vi "EllipseFitModule.vi"() -> ()   [LabVIEW 2011]
uses:
  Main/GlobalVariables.vi
panel:
  out "Valid Fit":bool
  in  "Reject Outliers":bool
  in  "bead":i32
  out "XY Graph bead 2":cluster{dbl[], dbl[]}[](graph)
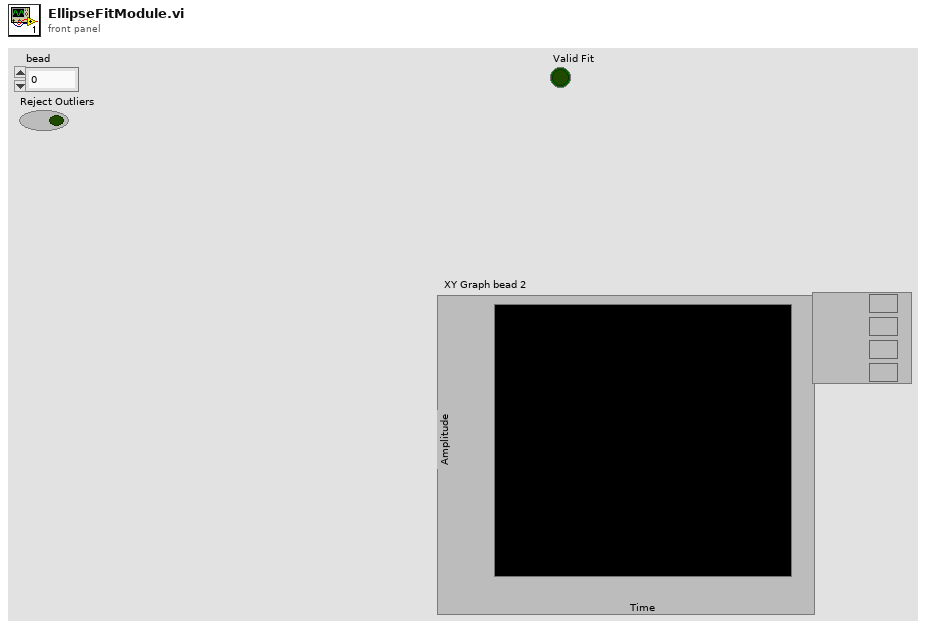
[diagram p1: front panel]
types:
  T1 = typedef "ResultManagerInstance.ctl" = cluster{"InstancePtr":u64}
  T2 = typedef "QTrkLocalizationResult.ctl" = cluster{"Queue Params":T3, "Position":T4, "Fast Estimate Position":cluster{"X":sgl, "Y":sgl}, "Error":i32, "Image mean":sgl}
  T3 = typedef "QTrkLocalizationJob.ctl" = cluster{"Frame#":u32, "Timestamp":u32, "ZLUT Index / bead#":i32, "Initial guess":T4}
  T4 = typedef "XYZf.ctl" = cluster{"X":sgl, "Y":sgl, "Z":sgl}
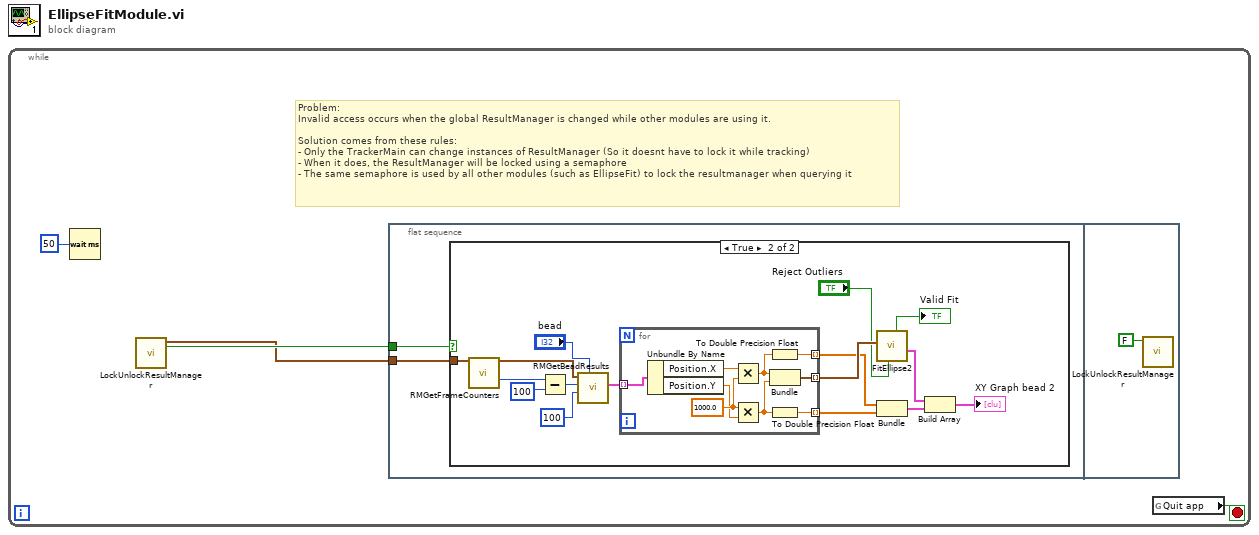
[diagram p0: block diagram]
diagram:
  n1 = while {
    stop <- w4 stop-if-true
    # "Problem: \nInvalid access occurs when the global ResultManager is changed while other modules are using it.\n\nSolution comes from these rules:\n- Only the TrackerMain can change instances of ResultManager (So it doesnt have to lock it while tracking)\n- When it does, the ResultManager will be locked using a semaphore\n- The same semaphore is used by all other modules (such as EllipseFit) to lock the resultmanager when querying it"
    n2 = Wait (ms)(milliseconds to wait=u32 50) -> ()  [unwired: 1 out]
    n3 = call "LockUnlockResultManager.vi"() -> ("Valid non-zero instance"=w2:bool, "ResultManager"=w1:T1)  [unwired: 9 in, 1 out]
    n4 = flat-sequence {
      tunnel: w2 -> [w6]
      tunnel: w1 -> [w5]
      frame #0 {
        n5 = case shown="True" w6 {
          tunnel: w5 -> [_ w22]
          frame False {
          }
          frame True {
            n6 = call "RMGetFrameCounters.vi"("ResultManager"=w22) -> ("ResultManager (out)"=w21:T1, "endFrame"=w20:i32)  [unwired: 7 in, 6 out]
            n7 = Subtract(x=w20, y=100) -> (x-y=w18:i32)
            n8 = call "RMGetBeadResults.vi"("bead"="bead", "numFrames"=100, "startFrame (0)"=w18, "ResultManager"=w21) -> ("results"=w15:T2[])  [unwired: 5 in, 2 out]
            n9 = for {
              tunnel: w15 -> [w31] mode=indexing
              tunnel: [w29] -> w14 mode=indexing
              tunnel: [w25] -> w7 mode=indexing
              tunnel: [w27] -> w8 mode=indexing
              w30 = sgl 1000.0 ("x")
              n10 = Unbundle By Name(w31) -> ("Position.X"=w26:sgl, "Position.Y"=w28:sgl)
              n11 = Multiply(x=w26, y=w30) -> (x*y=w24:sgl)
              n12 = Multiply(x=w30, y=w28) -> (x*y=w23:sgl)
              n13 = To Double Precision Float(number=w24) -> (double precision float=w25:dbl)
              n14 = Bundle(w24, w23) -> (w29:cluster{sgl, sgl})  [unwired: 1 in]
              n15 = To Double Precision Float(number=w23) -> (double precision float=w27:dbl)
            }
            n16 = call "FitEllipse2.vi"("Reject Outliers"="Reject Outliers", "Input data"=w14) -> ("XY Fit"=w11:cluster{dbl[], dbl[]}, "Valid Fit"=→"Valid Fit":bool)  [unwired: 7 in, 1 out]
            n17 = Bundle(w7, w8) -> (w10:cluster{dbl[], dbl[]})  [unwired: 1 in]
            n18 = Build Array(w11, w10) -> (→"XY Graph bead 2":cluster{dbl[], dbl[]}[])
          }
        }
      }
      frame #1 {
        n19 = call "LockUnlockResultManager.vi"("Lock? (T)"=FALSE) -> ()  [unwired: 8 in, 3 out]
      }
    }
    n20 = global read "GlobalVariables.vi" "Quit app"() -> (w4:bool)
  }
